vi "GEA2 Initialize.vi"(0 "Board Index":i32, 5 "Source Address":u8=228 format="%.0x", 11 "error in":errorcluster) -> (4 "GEA2 Reference Out":refnum<k24>, 8 "Board ID":string, 15 "error out":errorcluster)   [LabVIEW 2014, in "GEA2_Toolkit.lvlib"]
doc: "This VI uses .NET DLLs to initialize a GEA2 connection over USB. The output is a reference to the newly opened GEA2 connection."
uses:
  library/GEA2_Toolkit.lvlib
  C:/Automation/DLLs/PC Tools .NET/GeaCommunication.dll
  Automation/DLLs/PC Tools .NET/GeaCommunication.dll
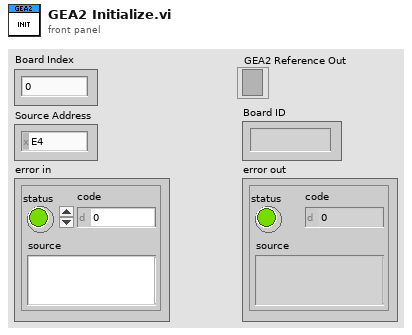
[diagram p1: front panel]
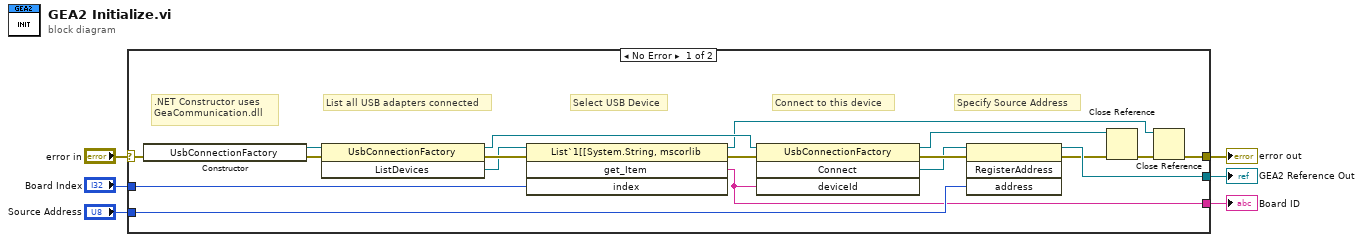
[diagram p0: block diagram]
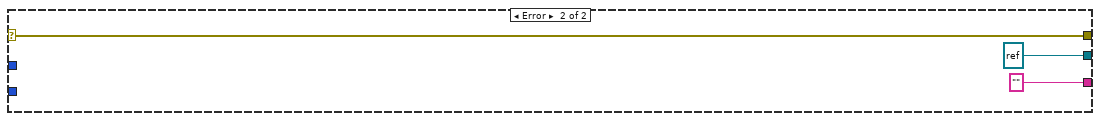
[diagram p2: hidden frame]
diagram:
  n1 = case shown="No Error" "error in" {
    selector: "error in" -> [w14 w27]
    tunnel: "Board Index" -> [w21 _]
    tunnel: [w7 w27] -> w6
    tunnel: [w18 refnum<k24> refnum ("Connect")] -> w4
    tunnel: "Source Address" -> [w16 _]
    tunnel: [w15 "" ("get_Item")] -> w1
    frame No Error {
      # "Specify Source Address"
      # "Connect to this device"
      # "Select USB Device"
      # "List all USB adapters connected"
      # ".NET Constructor uses\nGeaCommunication.dll"
      n2 = constructor class="UsbConnectionFactory"(error in=w14) -> (reference out=w10:refnum<k24>, error out=w13:errorcluster)  [unwired: 2 in, 1 out]
      n3 = invoke class="UsbConnectionFactory" method="ListDevices"(reference=w10, error in=w13) -> (reference out=w12:refnum<k24>, error out=w23:errorcluster, "ListDevices"=w22:refnum<k24>)  [unwired: 1 in]
      n4 = invoke class="List`1[[System.String, mscorlib" method="get_Item"(reference=w22, error in=w23, "index"=w21) -> (reference out=w9:refnum<k24>, error out=w24:errorcluster, "get_Item"=w15:string)  [unwired: 1 in, 1 out]
      n5 = invoke class="UsbConnectionFactory" method="Connect"(reference=w12, error in=w24, "deviceId"=w15) -> (reference out=w19:refnum<k24>, error out=w20:errorcluster, "Connect"=w11:refnum<k24>)  [unwired: 1 in, 1 out]
      n6 = invoke method="RegisterAddress"(reference=w11, error in=w20, "address"=w16) -> (reference out=w18:refnum<k24>, error out=w17:errorcluster)  [unwired: 1 in, 2 out]
      n7 = Close Reference(reference=w19, error in (no error)=w17) -> (error out=w8:errorcluster)
      n8 = Close Reference(reference=w9, error in (no error)=w8) -> (error out=w7:errorcluster)
    }
    frame Error {
    }
  }
  "error out" <- w6
  "GEA2 Reference Out" <- w4
  "Board ID" <- w1
